vi "PWM Out (subVI).vi"(1 "High Pulse":u16, 2 "Low Pulse":u16) -> (0 "PWM Output":bool)   [LabVIEW 2015]
doc: "This subVI supports a PWM output application. It translates the Low Pulse and High Pulse inputs to the number of milliseconds that the output PWM should stay low and high, respectively."
panel:
  # "This subVI supports a PWM output application.  It translates the Low Pulse and High Pulse inputs to the number of milliseconds that the output PWM should stay low and high, respectively."
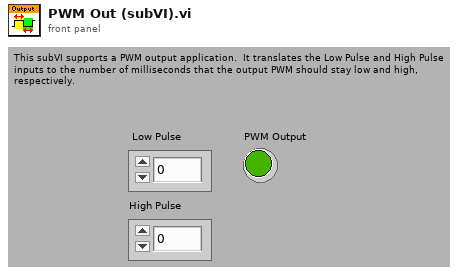
[diagram p1: front panel]
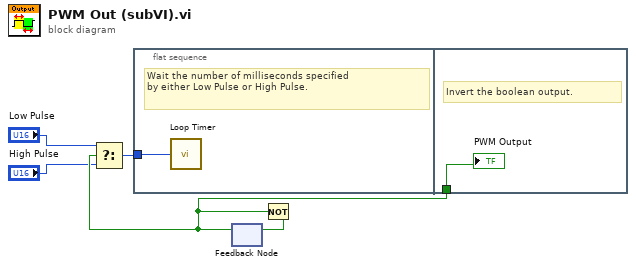
[diagram p0: block diagram]
diagram:
  n1 = flat-sequence {
    tunnel: w5 -> [w6]
    tunnel: w3 -> [w7]
    frame #0 {
      # "Wait the number of milliseconds specified\nby either Low Pulse or High Pulse."
      n2 = call "Loop Timer"("Count(mSec)"=w6) -> ()  [unwired: 1 out]
    }
    frame #1 {
      # "Invert the boolean output."
      "PWM Output" <- w7
    }
  }
  n3 = feedback #1() -> (w3:bool)  [unwired: 1 out]
  n4 = Select(t="Low Pulse", s=w3, f="High Pulse") -> (s? t:f=w5:u16)
  n5 = Not(x=w3) -> (.not. x?=w4:bool)
  n6 = feedback-in #1(w4) -> ()
